vi "StarWarsMelody2 (SubVI).vi"() -> (3 "Array":dbl[][](array[numeric]))   [LabVIEW 2014]
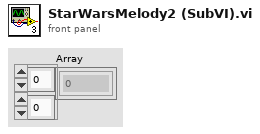
[diagram p1: front panel]
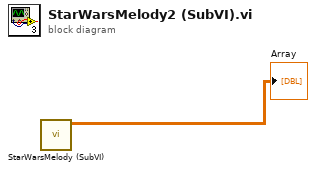
[diagram p0: block diagram]
diagram:
  n1 = call "StarWarsMelody (SubVI).vi"() -> ("Array"=→"Array":dbl[][])  [unwired: 11 in]
